vi "MAG STAB (MTDC).vi"(0 "MagQ":refnum<queue>, 5 "VISA In":refnum<visa-resource-name>, 7 "Boolean":bool, 11 "Error out":errorcluster, 12 "P-Mode Ramp Rate (A/s)":dbl) -> (4 "MagQ":refnum<queue>, 6 "VISA Out":refnum<visa-resource-name>, 15 "error out":errorcluster)   [LabVIEW 2025]
uses:
  <instrlib>/SMS LabVIEW Drivers/Source Code/Cryogenic Ltd SMSXXX.lvlib
  <instrlib>/SMS LabVIEW Drivers/Source Code/Public/PSU Status.ctl
panel:
  in  "PSU Status In":T1={"Ramp Target"=enum."ZERO", "Pause"=FALSE, "Switch Heater"=FALSE, "Persistent Field"=0.0, "Persistent Current"=0.0, "Tesla"=FALSE, "Output (T)"=0.0, "Output (A)"=0.0, "X Trip"=enum."DISABLED", "Ramp Rate (A/s)"=0.0, "V Limit (V)"=0.0, "Heater Voltage"=0.0, "MAX Setpoint (A)"=0.0, "MAX Setpoint (T)"=0.0, "MID Setpoint (A)"=0.0, "MID Setpoint (T)"=0.0, "Lock"=FALSE, "Field Constant"=0.0, "Remote"=FALSE, "Direction"=enum."POSITIVE", "Helium Level"=0, "Quench !"=FALSE, "Voltage"=0.0, "V Limit !"=FALSE, "Ramping"=FALSE, "At Target"=FALSE, "Trip Field"=0.0, "Trip Current"=0.0, "Current State"=enum."1. INIT MAG", "MAG Reference"="COM4"} {"Trip Current" format="%.3f"; "Trip Field" format="%.4f"; "Voltage" format="%.2f"; "Field Constant" format="%.6f"; "MID Setpoint (T)" format="%.4f"; "MID Setpoint (A)" format="%.3f"; "MAX Setpoint (T)" format="%.4f"; "MAX Setpoint (A)" format="%.3f"; "Heater Voltage" format="%.2f"; "V Limit (V)" format="%.2f"; "Ramp Rate (A/s)" format="%.3f"; "Output (A)" format="%.3f"; "Output (T)" format="%.4f"; "Persistent Current" format="%.3f"; "Persistent Field" format="%.4f"}
  out "PSU Status Out":T1={"Ramp Target"=enum."ZERO", "Pause"=FALSE, "Switch Heater"=FALSE, "Persistent Field"=0.0, "Persistent Current"=0.0, "Tesla"=FALSE, "Output (T)"=0.0, "Output (A)"=0.0, "X Trip"=enum."DISABLED", "Ramp Rate (A/s)"=0.0, "V Limit (V)"=0.0, "Heater Voltage"=0.0, "MAX Setpoint (A)"=0.0, "MAX Setpoint (T)"=0.0, "MID Setpoint (A)"=0.0, "MID Setpoint (T)"=0.0, "Lock"=FALSE, "Field Constant"=0.0, "Remote"=FALSE, "Direction"=enum."POSITIVE", "Helium Level"=0, "Quench !"=FALSE, "Voltage"=0.0, "V Limit !"=FALSE, "Ramping"=FALSE, "At Target"=FALSE, "Trip Field"=0.0, "Trip Current"=0.0, "Current State"=enum."1. INIT MAG", "MAG Reference"="COM4"} {"Trip Current" format="%.3f"; "Trip Field" format="%.4f"; "Voltage" format="%.2f"; "Field Constant" format="%.6f"; "MID Setpoint (T)" format="%.4f"; "MID Setpoint (A)" format="%.3f"; "MAX Setpoint (T)" format="%.4f"; "MAX Setpoint (A)" format="%.3f"; "Heater Voltage" format="%.2f"; "V Limit (V)" format="%.2f"; "Ramp Rate (A/s)" format="%.3f"; "Output (A)" format="%.3f"; "Output (T)" format="%.4f"; "Persistent Current" format="%.3f"; "Persistent Field" format="%.4f"}
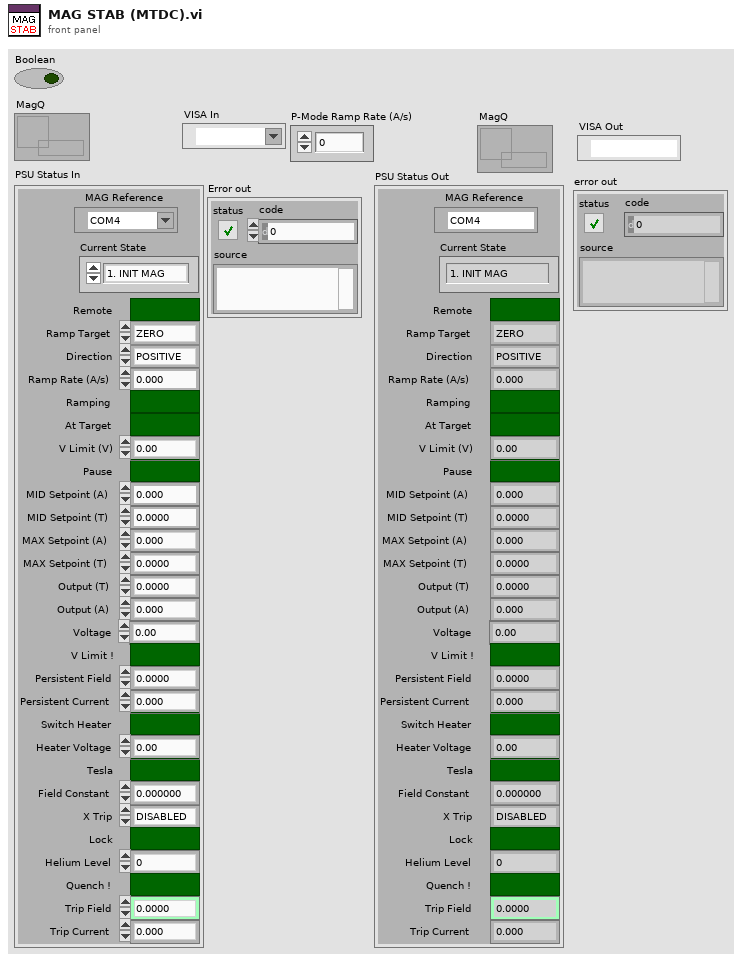
[diagram p1: front panel]
types:
  T1 = typedef "PSU Status.ctl" = cluster{"Ramp Target":enum16{"ZERO", "MID", "MAX"}, "Pause":bool, "Switch Heater":bool, "Persistent Field":dbl, "Persistent Current":dbl, "Tesla":bool, "Output (T)":dbl, "Output (A)":dbl, "X Trip":enum16{"DISABLED", "ENABLED", "ACTIVE"}, "Ramp Rate (A/s)":dbl, "V Limit (V)":dbl, "Heater Voltage":dbl, "MAX Setpoint (A)":dbl, "MAX Setpoint (T)":dbl, "MID Setpoint (A)":dbl, "MID Setpoint (T)":dbl, "Lock":bool, "Field Constant":dbl, "Remote":bool, "Direction":enum16{"POSITIVE", "NEGATIVE", "OPEN", "UNIPOLAR"}, "Helium Level":u16, "Quench !":bool, "Voltage":dbl, "V Limit !":bool, "Ramping":bool, "At Target":bool, "Trip Field":dbl, "Trip Current":dbl, "Current State":enum16{"1. INIT MAG", "2. MAG ON", "3. MAG_STAB", "4. MAG IDLE", "5. PREP NEXT FIELD", "6. APPLY NEXT FIELD", "7. PREP OFF", "8. MAG OFF (Reset)"}, "MAG Reference":refnum<visa-resource-name>}
  T2 = enum16{"1. INIT MAG", "2. MAG ON", "3. MAG_STAB", "4. MAG IDLE", "5. PREP NEXT FIELD", "6. APPLY NEXT FIELD", "7. PREP OFF", "8. MAG OFF (Reset)"}
  T3 = enum16{"RAMP TO ZERO", "RAMP TO MID", "RAMP TO MAX"}
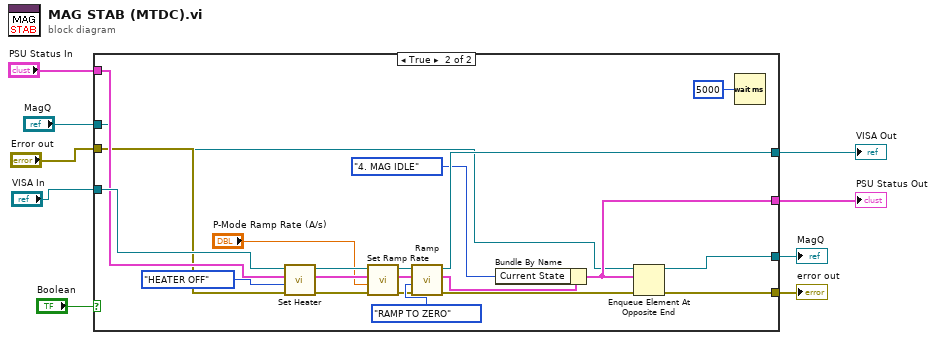
[diagram p0: block diagram]
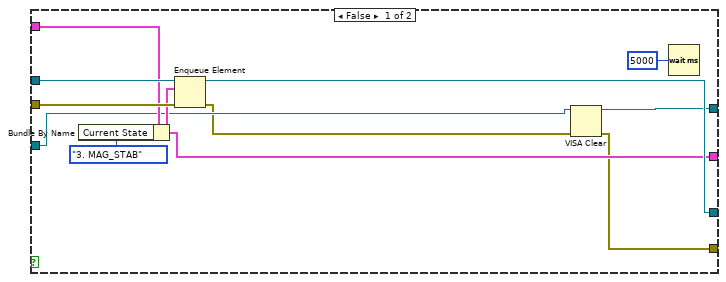
[diagram p2: hidden frame]
diagram:
  n1 = case shown="True" "Boolean" {
    tunnel: [w10 w21] -> w2
    tunnel: [w20 w40] -> w3
    tunnel: [w15 w34] -> w4
    tunnel: [w13 w37] -> w5
    tunnel: "VISA In" -> [w14 w33]
    tunnel: "PSU Status In" -> [w16 w32]
    tunnel: "Error out" -> [w17 w31]
    tunnel: "MagQ" -> [w18 w30]
    frame False {
      n2 = Bundle By Name(cluster=w16, "Current State"=T2."3. MAG_STAB") -> (w15:T1)
      n3 = Enqueue Element(queue=w18, element=w15, error in (no error)=w17) -> (queue out=w20:refnum<queue>, error out=w11:errorcluster)  [unwired: 1 in, 1 out]
      n4 = VISA Clear(VISA resource name=w14, error in (no error)=w11) -> (VISA resource name out=w13:refnum<visa-resource-name>, error out=w10:errorcluster)
      n5 = Wait (ms)(milliseconds to wait=u32 5000) -> ()  [unwired: 1 out]
    }
    frame True {
      n6 = call <instrlib>:"Set Heater.vi"("Error in (no error)"=w31, "Heater (On/Off)"=enum16{"HEATER OFF", "HEATER ON"}."HEATER OFF", "PSU Status In"=w32, "VISA Resource Name In"=w33) -> ("Error out"=w29:errorcluster, "PSU Status Out"=w27:T1, "VISA Resource Name Out"=w28:refnum<visa-resource-name>)  [unwired: 4 in, 1 out]
      n7 = call <instrlib>:"Set Ramp Rate.vi"("Error in (no error)"=w29, "Ramp Rate (A/s)"="P-Mode Ramp Rate (A/s)", "PSU Status In"=w27, "VISA Resource Name In"=w28) -> ("Error out"=w24:errorcluster, "PSU Status Out"=w26:T1, "VISA Resource Name Out"=w25:refnum<visa-resource-name>)  [unwired: 4 in, 1 out]
      n8 = call <instrlib>:"Ramp.vi"("Error in (no error)"=w24, "Ramp Target"=T3."RAMP TO ZERO", "PSU Status In"=w26, "VISA Resource Name In"=w25) -> ("Error out"=w36:errorcluster, "PSU Status Out"=w35:T1, "VISA Resource Name Out"=w37:refnum<visa-resource-name>)  [unwired: 4 in, 1 out]
      n9 = Bundle By Name(cluster=w35, "Current State"=T2."4. MAG IDLE") -> (w34:T1)
      n10 = Enqueue Element At Opposite End(queue=w30, element=w34, error in (no error)=w36) -> (queue out=w40:refnum<queue>, error out=w21:errorcluster)  [unwired: 1 in, 1 out]
      n11 = Wait (ms)(milliseconds to wait=u32 5000) -> ()  [unwired: 1 out]
    }
  }
  "VISA Out" <- w5
  "PSU Status Out" <- w4
  "MagQ" <- w3
  "error out" <- w2
